vi "Actor Core.vi"(8 "error in":errorcluster, 11 "CS++DSCTrendViewer in":refnum<class "CS++DSCTrendViewer.lvclass">) -> (0 "error out":errorcluster, 3 "Actor out":refnum<class "Actor.lvclass">)   [LabVIEW 2014, in "CS++DSCTrendViewer.lvlib" / "CS++DSCTrendViewer.lvclass"]
doc: "(<B>Filename</B>: Actor Framework.lvlib:Actor.lvclass:Actor Core.vi)\n\nReceives messages to the actor, reacts to them, and initiates any error handling that may shut the actor down.\n\nDescendant classes may override this VI to append parallel tasks for the actor to complete while it handles messages. Overrides use the Call Parent Method node."
uses:
  CS++DSCTrendViewer.lvclass
  <vilib>/ActorFramework/Actor/Actor.lvclass
  CS++DSCTrendViewer.lvclass/CS++DSCTrendViewer.ctl
  CSPP_Core/Actors/CS++BaseActor/CS++BaseActor.lvclass/CS++BaseActor.ctl
  CSPP_Core/Actors/CS++GUIActor/CS++GUIActor.lvclass/CS++GUIActor.ctl
  <vilib>/ActorFramework/Actor/Actor.lvclass/Actor.ctl
  <vilib>/ActorFramework/Message Enqueuer/Message Enqueuer.lvclass/Message Enqueuer.ctl
  CSPP_Core/Actors/CS++GUIActor/Read Stop-Event.vi
  CSPP_Core/Actors/CS++GUIActor/Read PV-Update.vi
  <vilib>/ActorFramework/Message Enqueuer/Init from Existing Queue.vi
  <vilib>/ActorFramework/Message Enqueuer/Enqueue.vi
  <vilib>/ActorFramework/Message Priority Queue/Priority Enqueue.vi
  CSPP_Core/Classes/CS++ProcessVariables/ProcessVariable/PV.lvclass
  <vilib>/ActorFramework/Message Enqueuer/Message Enqueuer.lvclass
  <vilib>/ActorFramework/Stop Msg/Stop Msg.lvclass
  CSPP_Core/Actors/CS++GUIActor/CS++GUIActor.lvclass
  CSPP_Core/Actors/CS++BaseActor/CS++BaseActor.lvclass
panel:
  in  "NIHyperTrend":refnum<k7>(container)
  in  "Stop Button":bool
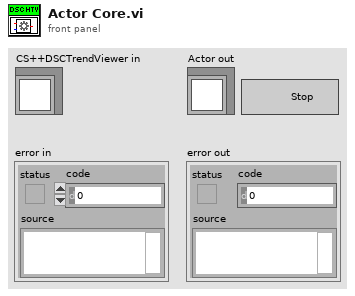
[diagram p1: front panel]
types:
  T1 = enum32{"Invalid", "Standard", "Closed", "Hidden", "Minimized", "Maximized"}
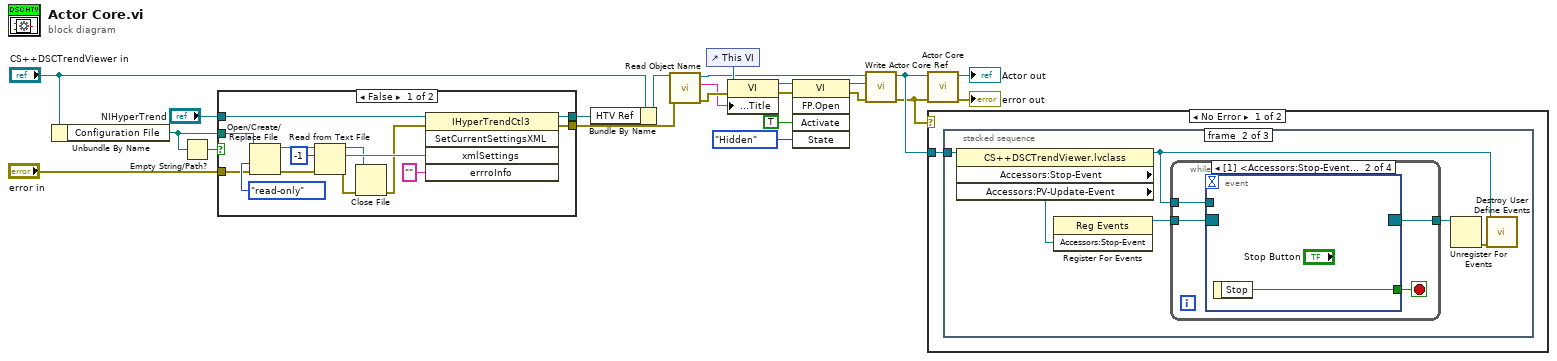
[diagram p0: block diagram]
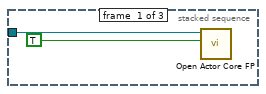
[diagram p3: hidden frame]
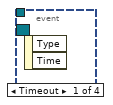
[diagram p4: hidden frame]
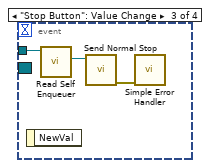
[diagram p5: hidden frame]
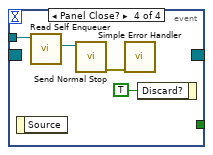
[diagram p6: hidden frame]
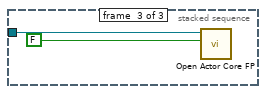
[diagram p7: hidden frame]
diagram:
  n1 = Unbundle By Name("CS++DSCTrendViewer in") -> ("Configuration File"=w18:path)
  n2 = Empty String/Path?(string/path=w18) -> (empty?=w19:bool)
  n3 = case shown="False" w19 {
    tunnel: "NIHyperTrend" -> [w27 w37]
    tunnel: "error in" -> [w26 w38]
    tunnel: [w25 w38] -> w4
    tunnel: w18 -> [w24 _]
    tunnel: [w23 w37] -> w15
    frame False {
      n4 = Open/Create/Replace File(file path (use dialog)=w24, error in=w26, access (0:read/write)=enum16{"read/write", "read-only", "write-only"}."read-only") -> (refnum out=w33:refnum<file>, error out=w34:errorcluster)  [unwired: 3 in, 1 out]
      n5 = Read from Text File(file (use dialog)=w33, count=-1, error in=w34) -> (refnum out=w30:refnum<file>, text=w32:string, error out=w29:errorcluster)  [unwired: 1 in, 1 out]
      n6 = Close File(refnum=w30, error in=w29) -> (error out=w28:errorcluster)  [unwired: 1 out]
      n7 = invoke on="Invoke Node" class="IHyperTrendCtl3" method="SetCurrentSettingsXML"(reference=w27, error in=w28, "xmlSettings"=w32, "errroInfo"="") -> (reference out=w23:refnum<k7>, error out=w25:errorcluster)  [unwired: 1 in, 3 out]
    }
    frame True {
    }
  }
  n8 = Bundle By Name(cluster="CS++DSCTrendViewer in", "HTV Ref"=w15) -> (w2:refnum<class "CS++DSCTrendViewer.lvclass">)
  n9 = call "Read Object Name.vi"("error in (no error)"=w4, "CS++BaseActor in"=w2) -> ("error out"=w5:errorcluster, "Object Name"=w3:string, "CS++BaseActor out"=w1:refnum<class "CS++DSCTrendViewer.lvclass">)  [unwired: 7 in]
  n10 = control-ref of="This VI"() -> (w7:refnum<vi>)
  n11 = property class="VI"(reference=w7, error in=w5, "Front Panel.Title"=w3) -> (reference out=w13:refnum<vi>, error out=w14:errorcluster)
  n12 = invoke class="VI" method="FP.Open"(reference=w13, error in=w14, "Activate"=TRUE ("Activate?"), "State"=T1."Hidden") -> (reference out=w11:refnum<vi>, error out=w12:errorcluster)  [unwired: 1 in, 3 out]
  n13 = call "Write Actor Core Ref.vi"("error in (no error)"=w12, "Actor Core Ref"=w11, "CS++BaseActor in"=w1) -> ("error out"=w6:errorcluster, "CS++BaseActor out"=w8:refnum<class "CS++DSCTrendViewer.lvclass">)  [unwired: 7 in]
  n14 = call-parent "Actor Core.vi"("error in"=w6, "CS++GUIActor in"=w8) -> ("error out"=→"error out":errorcluster, "Actor out"=→"Actor out":refnum<class "Actor.lvclass">)  [unwired: 8 in]
  n15 = case shown="No Error" w6 {
    tunnel: w8 -> [w39 _]
    frame No Error {
      n16 = stacked-sequence {
        tunnel: w39 -> [w41 w45 w61]
        frame #0 {
          n17 = call "Open Actor Core FP.vi"("Open FP (F)"=TRUE, "CS++BaseActor in"=w41) -> ()  [unwired: 8 in, 2 out]
        }
        frame #1 {
          n18 = property class="CS++DSCTrendViewer.lvclass" props=["Accessors:Stop-Event", "Accessors:PV-Update-Event"](reference=w45) -> (reference out=w44:refnum<class "CS++DSCTrendViewer.lvclass">, "Accessors:Stop-Event"=w42:refnum<user-event>)  [unwired: 1 in, 2 out]
          n19 = register-events(w42) -> (reference out=w43:refnum<event-registration>)  [unwired: 2 in, 1 out]
          n20 = while {
            tunnel: w43 -> [w51]
            tunnel: w44 -> [w50]
            tunnel: [w48] -> w47
            stop <- w49 stop-if-true
            n21 = event shown="[1] <Accessors:Stop-Event>: User Event" {
              selector: w51 -> [_ _ _ _]
              dyn-events: [_ _ _ _] -> w48
              timeout: _ -> [_ _ _ _]
              tunnel: w50 -> [_ _ w55 w59]
              tunnel: [_ w52 _ _] -> w49
              event Timeout {
                n22 = event-data() -> ()  [unwired: 1 in, 2 out]
              }
              event User Event {
                n23 = event-data() -> ("Stop"=w52:bool)  [unwired: 1 in]
              }
              event "Stop Button": Value Change {
                n24 = event-data() -> ()  [unwired: 1 in, 1 out]
                n25 = call <vilib>:"Read Self Enqueuer.vi"("Actor"=w55) -> ("Self Enqueuer"=w54:refnum<class "Message Enqueuer.lvclass">)  [unwired: 10 in]
                n26 = call <vilib>:"Send Normal Stop.vi"("Message Enqueuer"=w54) -> ("error out"=w53:errorcluster)  [unwired: 10 in]
                n27 = call <vilib>:"Simple Error Handler.vi"("error in (no error)"=w53) -> ()  [unwired: 4 in, 5 out]
              }
              event Panel Close? {
                n28 = event-data() -> ()  [unwired: 1 in, 1 out]
                n29 = call <vilib>:"Read Self Enqueuer.vi"("Actor"=w59) -> ("Self Enqueuer"=w58:refnum<class "Message Enqueuer.lvclass">)  [unwired: 10 in]
                n30 = call <vilib>:"Send Normal Stop.vi"("Message Enqueuer"=w58) -> ("error out"=w57:errorcluster)  [unwired: 10 in]
                n31 = call <vilib>:"Simple Error Handler.vi"("error in (no error)"=w57) -> ()  [unwired: 4 in, 5 out]
                n32 = event-data("Discard?"=TRUE) -> ()  [unwired: 1 in, 1 out]
              }
            }
          }
          n33 = Unregister For Events(event registration refnum=w47) -> (error out=w46:errorcluster)  [unwired: 1 in]
          n34 = call-dynamic "Destroy User Define Events.vi"("error in (no error)"=w46, "CS++GUIActor in"=w44) -> ()  [unwired: 8 in, 2 out]
        }
        frame #2 {
          n35 = call "Open Actor Core FP.vi"("Open FP (F)"=FALSE, "CS++BaseActor in"=w61) -> ()  [unwired: 8 in, 2 out]
        }
      }
    }
    frame Error {
    }
  }
